vi "VI Tester Menu Launch.vi"() -> ()   [LabVIEW 2013]
panel:
  out "Status":string
  out "Version":string
  # "© 2007 - 2019 JKI. All Rights Reserved."
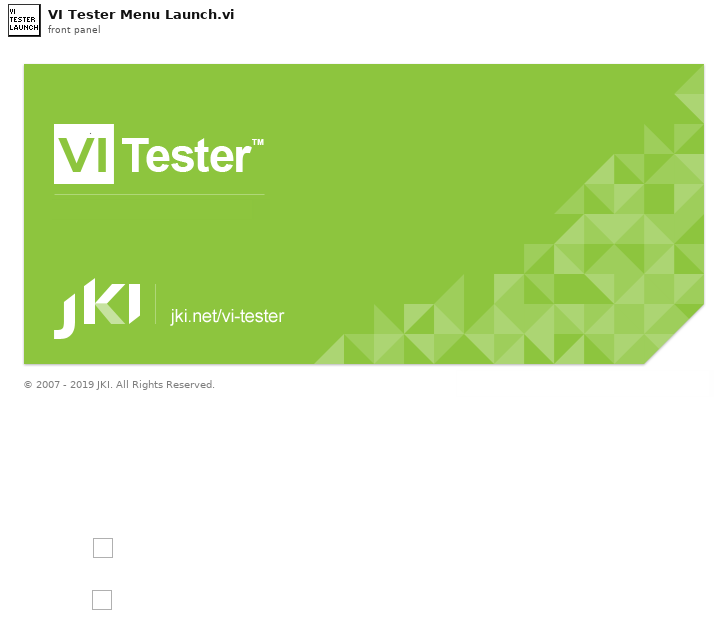
[diagram p1: front panel]
types:
  T1 = enum32{"Bad", "Idle", "Run top level", "Running"}
  T2 = typedef "Menu Launch Info - Cluster__jki_lib_application_control -- VI Tester.ctl" = cluster{"Application":refnum<vi>, "Selected Project Items":T3[]}
  T3 = typedef "Project Item Info - Cluster__jki_lib_application_control -- VI Tester.ctl" = cluster{"Type":string, "Name":string, "Path":path}
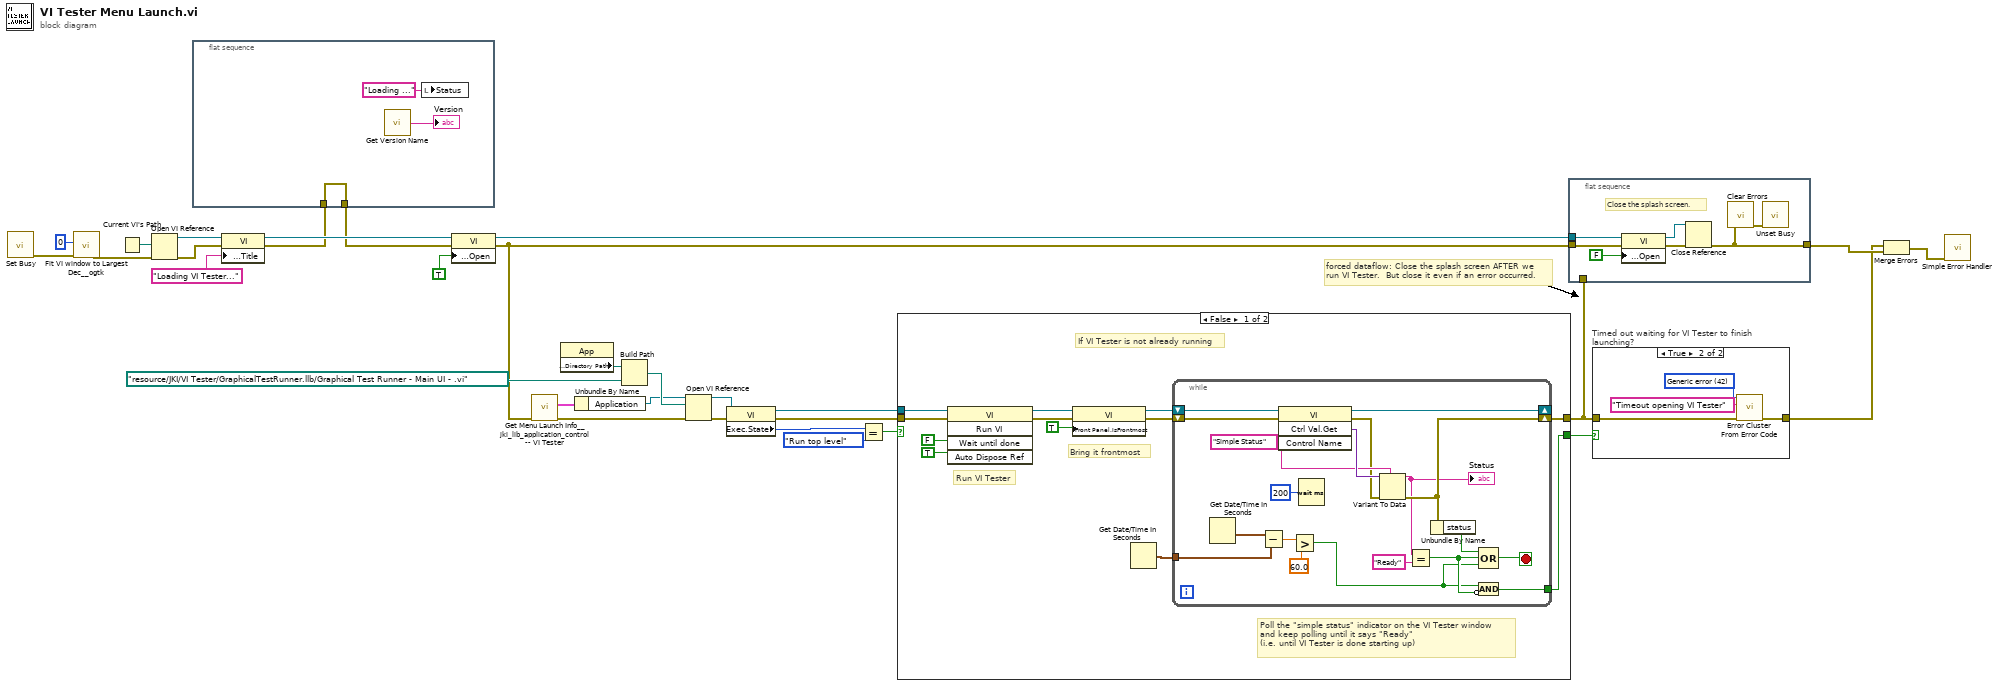
[diagram p0: block diagram]
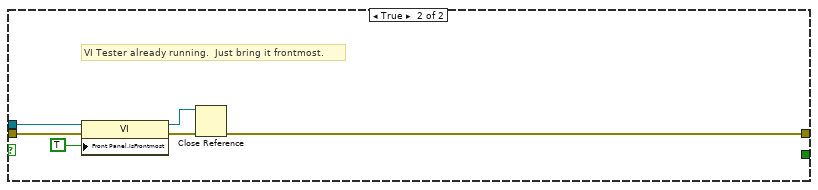
[diagram p3: hidden frame]
diagram:
  # "forced dataflow: Close the splash screen AFTER we\nrun VI Tester.  But close it even if an error occurred."
  n1 = call <vilib>:"Set Busy.vi"() -> ("error out"=w2:errorcluster)  [unwired: 10 in, 1 out]
  n2 = call <userlib>:"Fit VI window to Largest Dec__ogtk.vi"("error in (no error)"=w2, "border spacing (2 px)"=0) -> ("error out"=w21:errorcluster)  [unwired: 4 in, 1 out]
  n3 = Current VI's Path() -> (path=w24:path)
  n4 = Open VI Reference(vi path=w24, error in (no error)=w21) -> (vi reference=w7:refnum<vi>, error out=w8:errorcluster)  [unwired: 4 in]
  n5 = flat-sequence {
    tunnel: w4 -> [w32]
    tunnel: [w32] -> w3
    frame #0 {
      n6 = call "Get Version Name.vi"() -> ("Version Name"=→"Version":string)
      n7 = local write "Status"("Loading ..." ("Status")) -> ()
    }
  }
  n8 = property class="VI"(reference=w7, error in=w8, "Front Panel.Title"="Loading VI Tester..." ("Front Panel Window:Title")) -> (reference out=w6:refnum<vi>, error out=w4:errorcluster)
  n9 = property class="VI"(reference=w6, error in=w3, "Front Panel Window:Open"=TRUE) -> (reference out=w14:refnum<vi>, error out=w13:errorcluster)
  n10 = call "Get Menu Launch Info__jki_lib_application_control -- VI Tester.vi"("error in (no error)"=w13) -> ("error out"=w18:errorcluster, "Menu Launch info"=w17:T2)  [unwired: 9 in]
  n11 = property class="App"() -> ("Application:Directory Path"=w22:path)  [unwired: 2 in, 2 out]
  n12 = Unbundle By Name(w17) -> ("Application"=w19:refnum<vi>)
  n13 = Build Path(base path=w22, name or relative path=path "resource/JKI/VI Tester/GraphicalTestRunner.llb/Graphical Test Runner - Main UI - .vi" ("path")) -> (appended path=w30:path)
  n14 = Open VI Reference(application reference (local)=w19, vi path=w30, error in (no error)=w18) -> (vi reference=w15:refnum<vi>, error out=w26:errorcluster)  [unwired: 3 in]
  n15 = property class="VI"(reference=w15, error in=w26) -> (reference out=w16:refnum<vi>, error out=w25:errorcluster, "Exec.State"=w29:T1)
  n16 = Equal?(x=w29, y=T1."Run top level") -> (x = y?=w27:bool)
  n17 = case shown="False" w27 {
    tunnel: w25 -> [w46 w70]
    tunnel: w16 -> [w43 w71]
    tunnel: [w37 w66] -> w11
    tunnel: [w35 _] -> w12
    frame False {
      # "Poll the \"simple status\" indicator on the VI Tester window\nand keep polling until it says \"Ready\"\n(i.e. until VI Tester is done starting up)"
      # "If VI Tester is not already running"
      # "Bring it frontmost"
      # "Run VI Tester"
      n18 = invoke class="VI" method="Run VI"(reference=w43, error in=w46, "Wait until done"=FALSE ("Wait Until Done"), "Auto Dispose Ref"=TRUE ("Auto Dispose Reference")) -> (reference out=w41:refnum<vi>, error out=w40:errorcluster)  [unwired: 1 in, 3 out]
      n19 = property class="VI"(reference=w41, error in=w40, "Front Panel.IsFrontmost"=TRUE ("Front Panel Window:Is Frontmost")) -> (reference out=w36:refnum<vi>, error out=w38:errorcluster)
      n20 = Get Date/Time In Seconds() -> (seconds since 1Jan1904=w39:timestamp)
      n21 = while {
        shift-right: [w58] -> w37
        shift-left: w38 -> [w54]
        shift-right: [w63] -> _
        shift-left: w36 -> [w55]
        tunnel: w39 -> [w48]
        tunnel: [w50] -> w35
        stop <- w53 stop-if-true
        w64 = "Simple Status" ("Control Name")
        n22 = Get Date/Time In Seconds() -> (seconds since 1Jan1904=w61:timestamp)
        n23 = Subtract(x=w61, y=w48) -> (x-y=w60:dbl)
        n24 = invoke class="VI" method="Ctrl Val.Get"(reference=w55, error in=w54, "Control Name"=w64) -> (reference out=w63:refnum<vi>, error out=w62:errorcluster, "Get Control Value Variant"=w65:variant)  [unwired: 1 in, 1 out]
        n25 = Greater?(x=w60, y=60.0) -> (0:w51:bool)
        n26 = Wait (ms)(milliseconds to wait=u32 200) -> ()  [unwired: 1 out]
        n27 = Variant To Data(error in=w62, type=w64, Variant=w65) -> (data=w47:string, error out=w58:errorcluster)
        "Status" <- w47
        n28 = Equal?(x=w47, y="Ready") -> (x = y?=w52:bool)
        n29 = Unbundle By Name(w58) -> ("status"=w57:bool)
        n30 = Compound Arithmetic op=OR(w57, w52, w51) -> (w53:bool)
        n31 = Compound Arithmetic op=AND(w51, invert w52) -> (w50:bool)
      }
    }
    frame True {
      # "VI Tester already running.  Just bring it frontmost."
      n32 = property class="VI"(reference=w71, error in=w70, "Front Panel.IsFrontmost"=TRUE ("Front Panel Window:Is Frontmost")) -> (reference out=w68:refnum<vi>, error out=w67:errorcluster)
      n33 = Close Reference(reference=w68, error in (no error)=w67) -> (error out=w66:errorcluster)
    }
  }
  n34 = flat-sequence {
    tunnel: w14 -> [w76]
    tunnel: [w72] -> w10
    tunnel: w11 -> [_]
    tunnel: w13 -> [w74]
    frame #0 {
      # "Close the splash screen."
      n35 = property class="VI"(reference=w76, error in=w74, "Front Panel Window:Open"=FALSE) -> (reference out=w77:refnum<vi>, error out=w75:errorcluster)
      n36 = Close Reference(reference=w77, error in (no error)=w75) -> (error out=w72:errorcluster)
      n37 = call <vilib>:"Clear Errors.vi"("error in (no error)"=w72) -> ("error out"=w73:errorcluster)  [unwired: 6 in]
      n38 = call <vilib>:"Unset Busy.vi"("error in (no error)"=w73) -> ()  [unwired: 10 in, 1 out]
    }
  }
  n39 = case "Timed out waiting for VI Tester to finish launching?" shown="True" w12 {
    tunnel: w11 -> [w79 w81]
    tunnel: [w79 w80] -> w9
    frame False {
    }
    frame True {
      w83 = 42 items=["No error", "Argument error", "Memory is full", "Out of zone", "End of file", "File already open", "Generic file I/O error", "File not found", "File permission error", "Disk is full", "Duplicate path", "Too many files open", "System feature not enabled", "Resource file not found", "Cannot add resource", "Resource not found", "Image not found", "Image memory error", "Pen does not exist", "Config type invalid", "Config token not found", "Config parse error", "Config memory error", "Bad external code format", "Bad external code offset", "External code not present", "Null window", "Destroy window error", "Null menu", "Print aborted", "Bad print record", "Print driver error", "Windows error during printing", "Memory error during printing", "Print dialog error", "Generic print error", "Invalid device refnum", "Device not found", "Device parameter error", "Device unit error", "Cannot open device", "Device call aborted", "Generic error", "Cancelled by user", "Object ID too low", "Object ID too high", "Object not in heap", "Unknown heap", "Unknown object (invalid DefProc)", "Unknown object (DefProc not in table)", "Message out of range", "Invalid (null) method", "Unknown message", "Manager call not supported", "Bad address", "Network operation in progress", "Network operation timed out", "Connection is busy", "Network attribute not supported", "Network error", "Address in use", "System out of memory", "Connection aborted", "Connection refused", "Not connected", "Already connected", "Connection closed", "Initialization error (interapplication manager)", "Bad occurrence", "Wait on unbound occurrence handler", "Occurrence queue overflow", "Datalog type conflict", "Unused", "Unrecognized type (interapplication manager)", "Memory corrupt", "Failed to make temporary DLL", "Old CIN version", "Drag socket not found", "Failed to load drop-object", "Failed to register OLE object", "Failed to release OLE object", "Format specifier type mismatch", "Unknown format specifier", "Too few format specifiers", "Too many format specifiers", "Scan failed", "Newer CIN version", "Error converting to variant", "Runtime menu error", "Password tampered", "Variant attribute not found", "Incompatible variant data type", "Event data is not available", "Event Store is not present", "Occurrence is not found", "Event Queue is not created", "Event info is not available", "Refnum passed is NULL", "Error retrieving Class GUID", "Error retrieving CoClass GUID", "Error retrieving TypeLib GUID.", "Bad built application magic bytes.", "Specific driver is different from the specific driver associated with the Logical Name.", "There is no session opened to the class driver.", "Max Error", "MAX - Error with config objects", "MAX - Error loading configuration", "MAX - Group not supported"]
      n40 = call <vilib>:"Error Cluster From Error Code.vi"("error in (no error)"=w81, "error message (\"\")"="Timeout opening VI Tester" ("error message (\"\")"), "error code (0)"=w83) -> ("error out"=w80:errorcluster)  [unwired: 6 in]
    }
  }
  n41 = Merge Errors(w9, w10) -> (w1:errorcluster)
  n42 = call <vilib>:"Simple Error Handler.vi"("error in (no error)"=w1) -> ()  [unwired: 4 in, 5 out]
